vi "Atto DRY Interface get Turbopump Frequency.vi"(8 "error in (no error)":errorcluster, 11 "TurbopumpFrequencyHz":u16) -> (0 "error out":errorcluster, 2 "function return":i32, 3 "TurbopumpFrequencyHz out":u16)   [LabVIEW 2016, in "attoDRYLib.lvlib"]
doc: "int32_t __cdecl AttoDRY_Interface_getTurbopumpFrequency(\n uint16_t *TurbopumpFrequencyHz);"
uses:
  <userlib>/attoDRYLib/attoDRYLib.lvlib
  <userlib>/attoDRYLib/attoDRYLib.dll
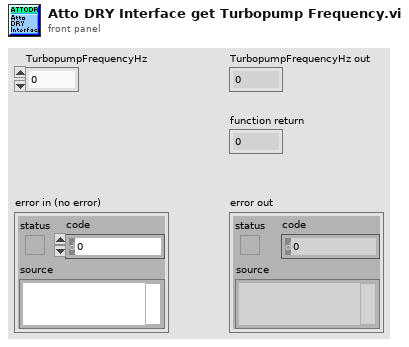
[diagram p1: front panel]
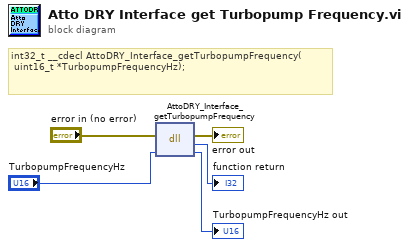
[diagram p0: block diagram]
diagram:
  # "int32_t __cdecl AttoDRY_Interface_getTurbopumpFrequency(\n\tuint16_t *TurbopumpFrequencyHz);"
  n1 = dll-call lib="C:/Program Files (x86)/National Instruments/LabVIEW 2016/user.lib/attoDRYLib/attoDRYLib.*" fn="AttoDRY_Interface_getTurbopumpFrequency"(error in="error in (no error)", "TurbopumpFrequencyHz"="TurbopumpFrequencyHz") -> (error out=→"error out":errorcluster, →"function return":i32, "TurbopumpFrequencyHz"=→"TurbopumpFrequencyHz out":u16)  [unwired: 2 in, 1 out]
